vi "Destroy.vi"(0 "reference in":refnum<class "Simulated-PowerModule.lvclass">, 11 "Error In":errorcluster) -> (4 "reference out":refnum<class "Simulated-PowerModule.lvclass">, 15 "Error Out":errorcluster)   [LabVIEW 2023, in "Simulated-PowerModule.lvlib" / "Simulated-PowerModule.lvclass"]
uses:
  Simulated-PowerModule.lvclass
  <vilib>/addons/_JKI.lib/Serialization/JSON/JKI JSON Serialization.lvlib
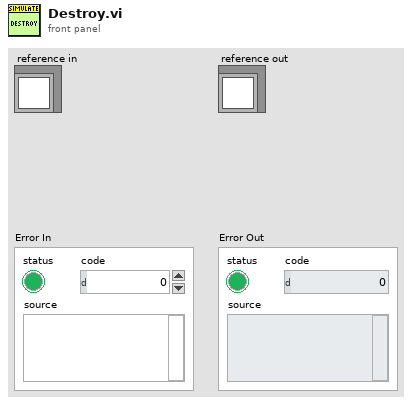
[diagram p1: front panel]
types:
  T1 = typedef "Simulated-PowerModule.lvlib/Simulated-PowerModule.lvclass/ObjectAttributes.ctl" = cluster{"JSON Config Path":path, "mode":T2, "Configuration":T3, "connected":bool, "reserved":bool, "energized":bool, "output enabled":bool, "setpoint":cluster{"voltage":dbl, "current":dbl, "resistance":dbl}, "last timestamp":i64, "measurement array":T6[], "profile":dbl[][], "step dt":i64}
  T2 = typedef "Simulated-PowerModule.lvlib/Simulated-PowerModule.lvclass/Mode.ctl" = u16
  T3 = typedef "Simulated-PowerModule.lvlib/Simulated-PowerModule.lvclass/Configuration.ctl" = cluster{"range":T4, "Limits":T5, "measurement array size":u32}
  T4 = typedef "PowerModuleInterface.lvlibp/PowerModuleInterface.lvclass/Range.ctl" = cluster{"Current Max (A)":dbl, "Current Min (A)":dbl, "Voltage Max (V)":dbl, "Voltage Min (V)":dbl}
  T5 = typedef "PowerModuleInterface.lvlibp/PowerModuleInterface.lvclass/Limits.ctl" = cluster{"Current Max (A)":dbl, "Current Min (A)":dbl, "Voltage Max (V)":dbl, "Voltage Min (V)":dbl, "Power Max (W)":dbl, "Power Min (W)":dbl}
  T6 = typedef "PowerModuleInterface.lvlibp/PowerModuleInterface.lvclass/Measurements.ctl" = cluster{"measured voltage (V)":dbl, "measured current (A)":dbl, "setpoint voltage (V)":dbl, "setpoint current (A)":dbl, "timestamp":dbl}
  T7 = enum16{"open", "replace", "create", "open or create", "replace or create", "replace or create with confirmation"}
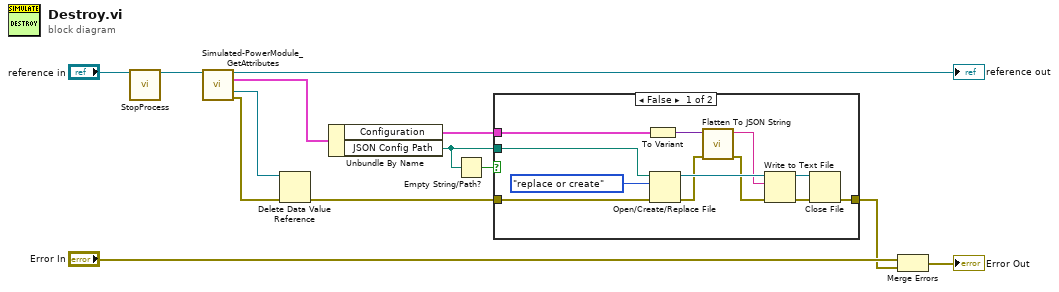
[diagram p0: block diagram]
diagram:
  n1 = call "StopProcess.vi"("reference in"="reference in") -> ("reference out"=w10:refnum<class "Simulated-PowerModule.lvclass">)  [unwired: 17 in, 1 out]
  n2 = call "Simulated-PowerModule_GetAttributes.vi"("reference in"=w10) -> ("reference out"=→"reference out":refnum<class "Simulated-PowerModule.lvclass">, "Data"=w1:T1, "DataRef"=w8:refnum<data-value>, "Error Out"=w9:errorcluster)  [unwired: 11 in]
  n3 = Delete Data Value Reference(data value reference=w8, error in=w9) -> (error out=w6:errorcluster)  [unwired: 1 out]
  n4 = Unbundle By Name(w1) -> ("Configuration"=w5:T3, "JSON Config Path"=w3:path)
  n5 = Empty String/Path?(string/path=w3) -> (empty?=w2:bool)
  n6 = case shown="False" w2 {
    tunnel: w6 -> [w24 w26]
    tunnel: w5 -> [w20 _]
    tunnel: [w15 w26] -> w4
    tunnel: w3 -> [w14 _]
    frame False {
      n7 = To Variant(anything=w20) -> (Variant=w19:variant)
      n8 = Open/Create/Replace File(file path (use dialog)=w14, error in=w24, operation (0:open)=T7."replace or create") -> (refnum out=w23:refnum<file>, error out=w22:errorcluster)  [unwired: 3 in, 1 out]
      n9 = call <vilib>:"Flatten To JSON String.vi"("error in"=w22, "Variant"=w19) -> ("error out"=w21:errorcluster, "JSON String"=w18:string)  [unwired: 8 in]
      n10 = Write to Text File(file (use dialog)=w23, text=w18, error in=w21) -> (refnum out=w16:refnum<file>, error out=w17:errorcluster)  [unwired: 1 in, 1 out]
      n11 = Close File(refnum=w16, error in=w17) -> (error out=w15:errorcluster)  [unwired: 1 out]
    }
    frame True {
    }
  }
  n12 = Merge Errors("Error In", w4) -> (→"Error Out":errorcluster)
